vi "Read Response.vi"(8 "error in (no error)":errorcluster, 11 "VISA resource name in":refnum<visa-resource-name>) -> (0 "error out":errorcluster, 2 "Response":string, 3 "VISA resource name":refnum<visa-resource-name>)   [LabVIEW 2020, in "CTI-Visa.lvlib"]
uses:
  CTI-Visa.lvlib
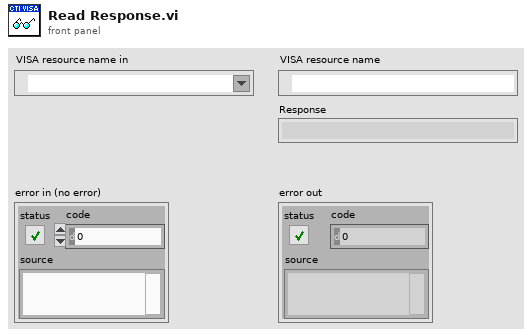
[diagram p1: front panel]
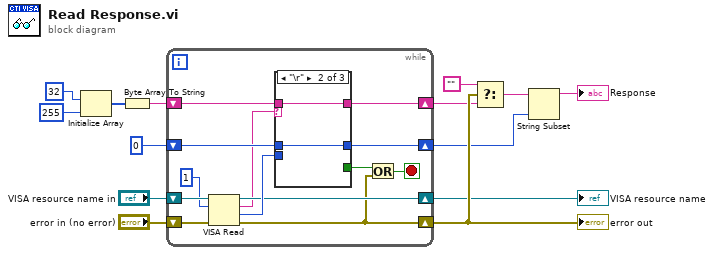
[diagram p0: block diagram]
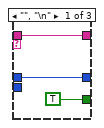
[diagram p2: hidden frame]
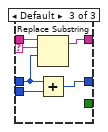
[diagram p3: hidden frame]
diagram:
  n1 = Initialize Array(u8 32 ("element"), 255 ("dimension size")) -> (w9:u8[])
  n2 = Byte Array To String(unsigned byte array=w9) -> (string=w8:string)
  n3 = while {
    shift-right: [w17] -> w14
    shift-left: "error in (no error)" -> [w26]
    shift-right: [w18] -> w6
    shift-left: "VISA resource name in" -> [w27]
    shift-right: [w21] -> w5
    shift-left: w8 -> [w24]
    shift-right: [w22] -> w1
    shift-left: 0 -> [w23]
    stop <- w19 stop-if-true
    n4 = VISA Read(VISA resource name=w27, byte count=u32 1, error in (no error)=w26) -> (VISA resource name out=w18:refnum<visa-resource-name>, read buffer=w16:string, return count=w20:u32, error out=w17:errorcluster)
    n5 = case shown="\"\\r\"" w16 {
      selector: w16 -> [_ _ w33]
      tunnel: w24 -> [w30 w32 w38]
      tunnel: w23 -> [w29 w31 w37]
      tunnel: [w29 w31 w36] -> w22
      tunnel: [w30 w32 w35] -> w21
      tunnel: w20 -> [_ _ w34]
      tunnel: [TRUE _ _] -> w15
      frame "", "\n" {
      }
      frame "\r" {
      }
      frame Default {
        n6 = Replace Substring(3:w37, 4:w33, 5:w38) -> (1:w35:string)  [unwired: 1 in, 1 out]
        n7 = Add(x=w37, y=w34) -> (x+y=w36:u32)
      }
    }
    n8 = Or(x=w15, y=w17) -> (x .or. y?=w19:bool)
  }
  "VISA resource name" <- w6
  "error out" <- w14
  n9 = Select(t="", s=w14, f=w5) -> (s? t:f=w3:string)
  n10 = String Subset(string=w3, length (rest)=w1) -> (substring=→"Response":string)  [unwired: 1 in]
